vi "sim.vi"() -> ()   [LabVIEW 2011]
uses:
  <vilib>/robotics/Simulator/NI_Robotics_Simulator.lvlib
  <vilib>/robotics/Starter Kit/1.0/Sim Host Interface/NI_Robotics_Starter Kit Host_Sim_1.0.lvclass
  <vilib>/Analysis/NI_AALPro.lvlib
  <vilib>/Analysis/7linalg.llb/Real Transpose Matrix.vi
  <vilib>/Analysis/Matrix/NI_Matrix.lvlib
  <vilib>/robotics/Starter Kit/Host Interface/NI_Robotics_Starter Kit Host.lvclass
  <vilib>/Analysis/NI_AALBase.lvlib
  <vilib>/Platform/TimedLoop/XDataNode/XDataNode.xnode
  <vilib>/Platform/TimedLoop/XDataNode/timing_clust.ctl
  <vilib>/Platform/TimedLoop/XDataNode/XDNodeRunTimeDep.lvlib
  <vilib>/Platform/TimedLoop/XDataNode/wakeup.ctl
  <vilib>/Platform/TimedLoop/XDataNode/nitl_modes.ctl
  <vilib>/Analysis/baseanly.llb/Real A x B.vi
  <vilib>/Analysis/Matrix/Numeric/Conversions/Array To Matrix - RA.vi
panel:
  in  "q":dbl step=0.01
  in  "K_ W":dbl step=0.01
  in  "K_ VL":dbl step=0.01
  in  "Paso":dbl
  in  "Tiempo":dbl
  in  "stop":bool
  out "X-Y":cluster{ext[], ext[]}(graph)
  out "VL":cluster{i32[], dbl[]}(graph)
  out "W":cluster{i32[], dbl[]}(graph)
  out "theta":cluster{i32[], ext[]}(graph)
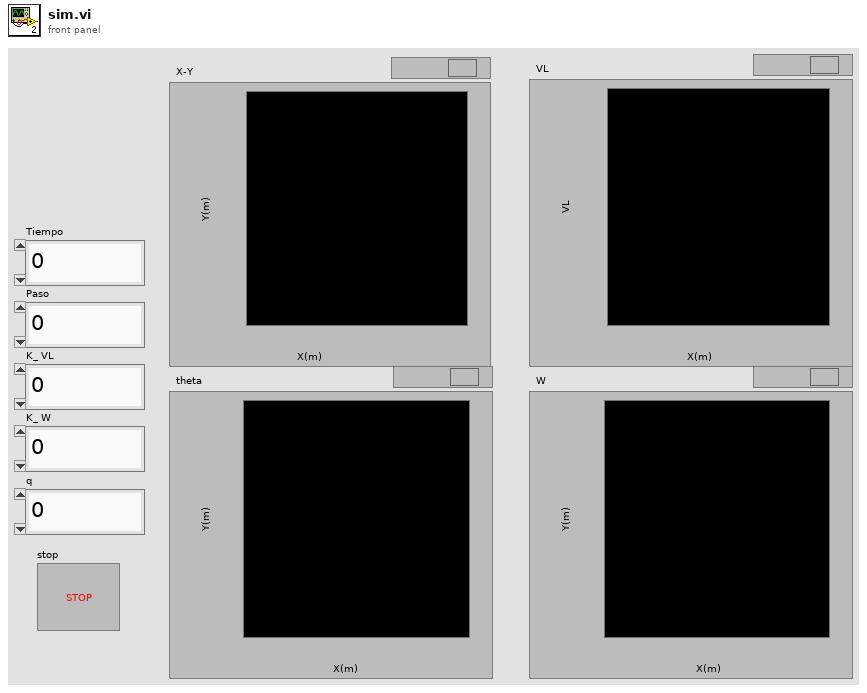
[diagram p1: front panel]
types:
  T1 = typedef "NI_Matrix.lvlib/RealMatrix.ctl" = dbl[][]
  T2 = typedef "XDNodeRunTimeDep.lvlib/timing_clust.ctl" = cluster{"Expected End [f-1]":u64, "Actual End [f-1]":u64, "Finished Late? [f-1]":bool, "Expected End [i-1]":u64, "Actual End [i-1]":u64, "Finished Late? [i-1]":bool, "Expected Start [i]":u64, "Actual Start [i]":u64, "Expected Start [f]":u64, "Actual Start [f]":u64, "Source Name":string, "Structure Name":string, "Period":i64, "Deadline":i64, "Offset":i64, "Start":i64, "Priority":i32, "Timeout":i32, "Mode":T3, "Wakeup Reason":T4, "Error":errorcluster, "Source Type":string, "Secondary Source Type":string, "Global End Time":u64, "Global Start Time":u64, "Frame Duration":u64, "Iteration Duration":u64, "Assigned CPU":i32, "I/O Scan Engine Mode":u32}
  T3 = typedef "XDNodeRunTimeDep.lvlib/nitl_modes.ctl" = enum32{"No Change", "Process missed periods, maintain original phase", "Discard missed periods, maintain original phase", "Process missed periods, ignore original phase", "Discard missed periods, ignore original phase"}
  T4 = typedef "XDNodeRunTimeDep.lvlib/wakeup.ctl" = enum32{"Normal", "Aborted", "Asynchronous wakeup", "Timing source error", "Timed loop error", "Timeout"}
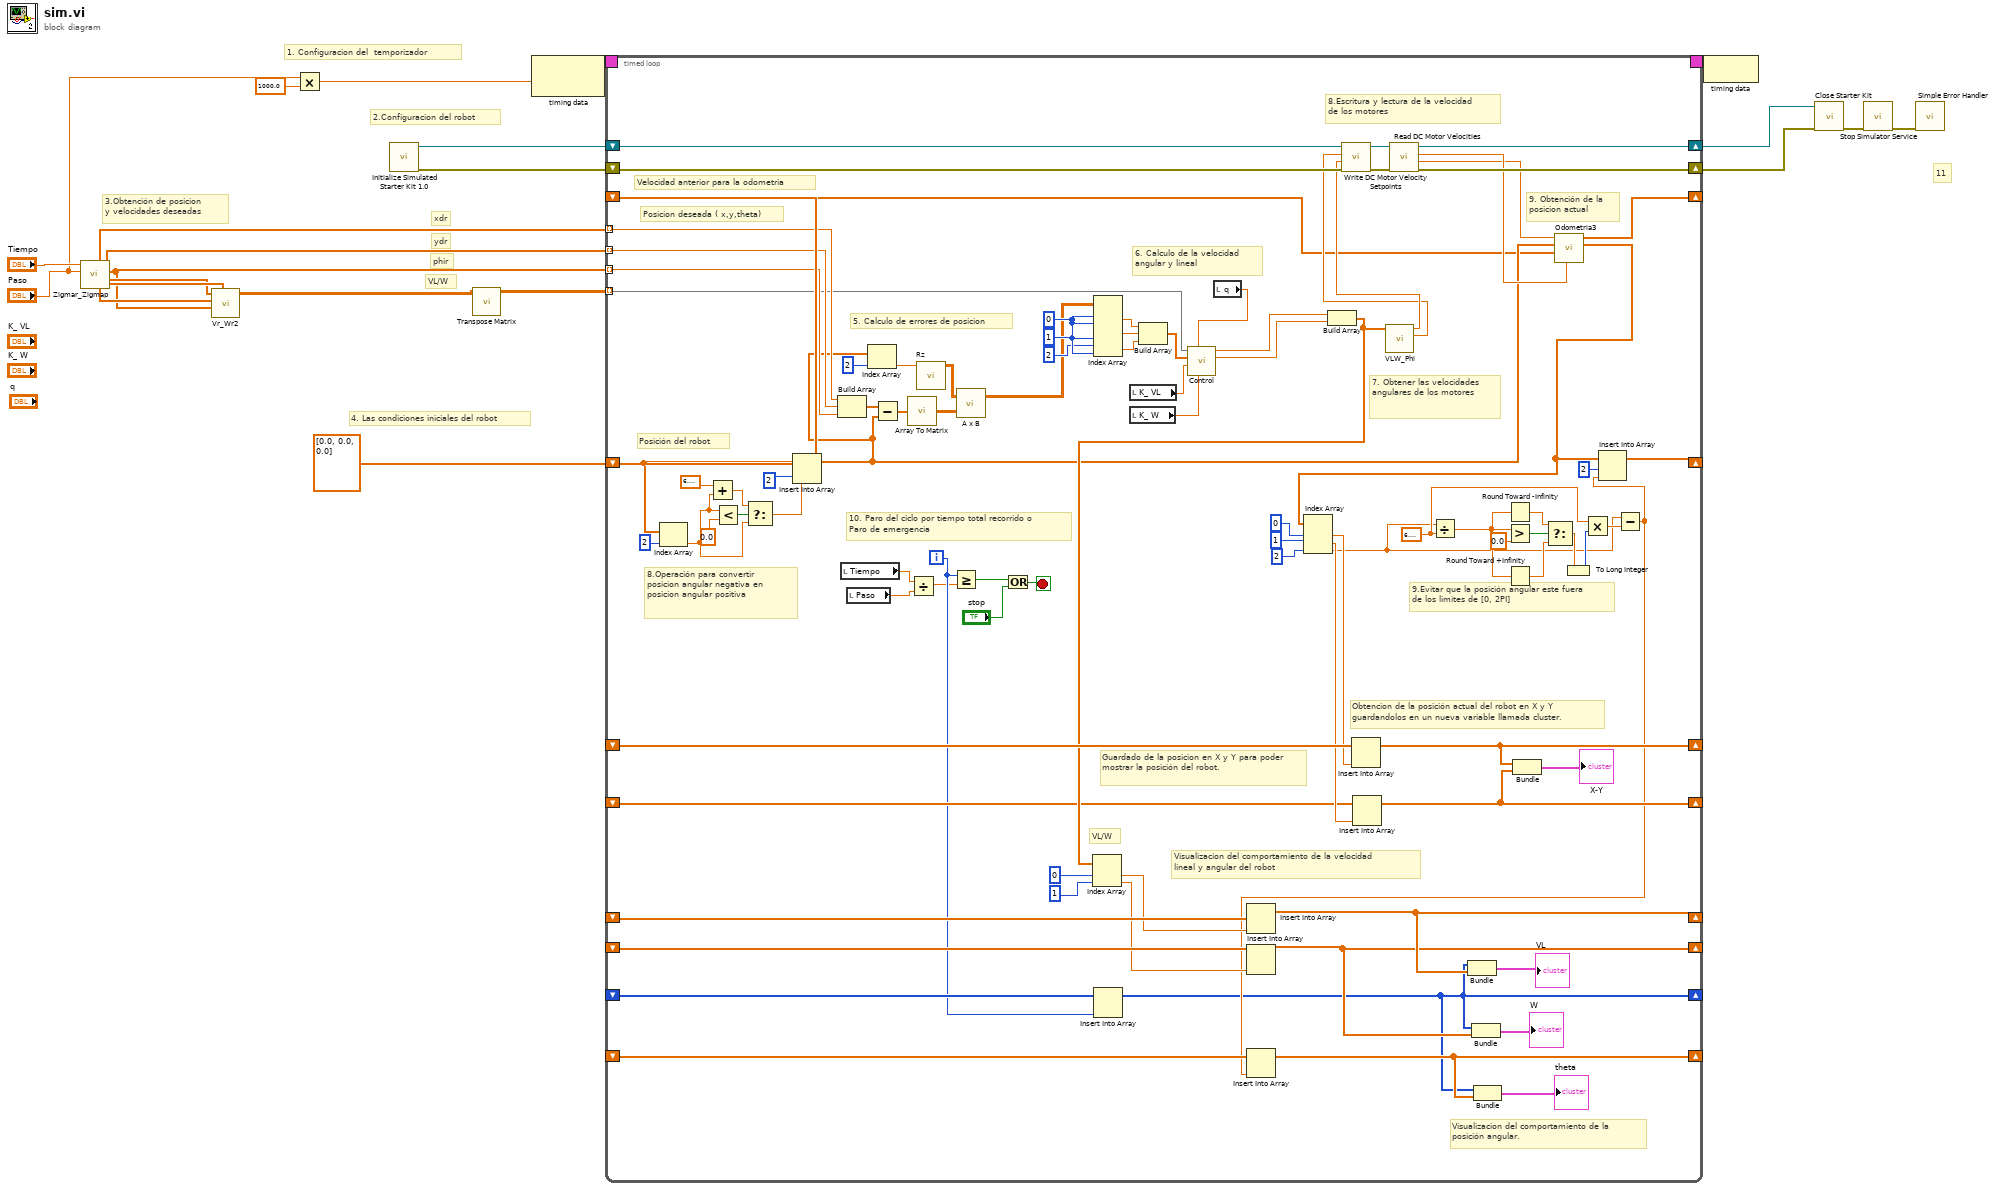
[diagram p0: block diagram]
diagram:
  w8 = dbl[] [0.0, 0.0, 0.0]
  # "4. Las condiciones iniciales del robot"
  # "VL/W"
  # "3.Obtención de posicion \ny velocidades deseadas"
  # "2.Configuracion del robot"
  # "1. Configuracion del  temporizador"
  # "phir"
  # "ydr"
  # "xdr"
  # "11"
  n1 = call "Zigmar_Zigmap.vi"("Paso"="Paso", "Tiempo"="Tiempo") -> ("Xdrp"=w16:dbl[], "Phir"=w14:dbl[], "Ydr"=w18:dbl[], "Ydrp"=w15:dbl[], "Xdr"=w13:dbl[], "Phirp"=w17:dbl[])  [unwired: 4 in]
  n2 = call "Vr_Wr2.vi"("Phirp"=w17, "Phir"=w14, "Ydrp"=w15, "Xdrp"=w16) -> ("VLW"=w2:T1)  [unwired: 7 in]
  n3 = Multiply(x="Paso", y=1000.0) -> (x*y=w5:dbl)
  n4 = call <vilib>:"Initialize Simulated Starter Kit 1.0.vi"() -> ("error out"=w4:errorcluster, "simulated starter kit host 1.0 out"=w3:refnum<class "NI_Robotics_Starter Kit Host_Sim_1.0.lvclass">)  [unwired: 10 in]
  n5 = call-poly <vilib>:"Transpose Matrix.vi"("Input Matrix"=w2) -> ("Matrix Transpose"=w1:T1)  [unwired: 9 in, 1 out]
  n6 = node-c288(w5) -> (w21:T2)
  n7 = timed-loop {
    shift-right: [w101] -> w9
    shift-left: w3 -> [w103]
    shift-right: [w100] -> w10
    shift-left: w4 -> [w102]
    timing: w21 -> [_]
    timing-out: [_] -> w20
    tunnel: w13 -> [w113] mode=indexing
    tunnel: w18 -> [w112] mode=indexing
    tunnel: w14 -> [w111] mode=indexing
    shift-right: [w89] -> _
    shift-left: w8 -> [w38]
    shift-right: [w37] -> _
    shift-left: w8 -> [w33]
    shift-right: [w93] -> _
    shift-left: _ -> [w98]
    shift-right: [w92] -> _
    shift-left: _ -> [w51]
    shift-right: [w68] -> _
    shift-left: _ -> [w77]
    shift-right: [w65] -> _
    shift-left: _ -> [w72]
    shift-right: [w62] -> _
    shift-left: _ -> [w67]
    shift-right: [w64] -> _
    shift-left: _ -> [w66]
    tunnel: w1 -> [w25] mode=indexing
    i -> [w50]
    stop <- w108 stop-if-true
    w60 = 0 ("index (col)")
    w88 = 6.283185307179586
    # "Visualizacion del comportamiento de la\nposición angular."
    # "Visualizacion del comportamiento de la velocidad \nlineal y angular del robot"
    # "VL/W"
    # "Obtencion de la posición actual del robot en X y Y\nguardandolos en un nueva variable llamada cluster."
    # "Guardado de la posicion en X y Y para poder mostrar la posición del robot."
    # "Posicion deseada ( x,y,theta)"
    # "10. Paro del ciclo por tiempo total recorrido o\nParo de emergencia"
    # "9.Evitar que la posición angular este fuera\nde los limites de [0, 2PI]"
    # "8.Operación para convertir posicion angular negativa en posicion angular positiva"
    # "Posición del robot"
    # "9. Obtención de la\nposicion actual"
    # "7. Obtener las velocidades\nangulares de los motores"
    # "6. Calculo de la velocidad \nangular y lineal"
    # "5. Calculo de errores de posicion"
    # "8.Escritura y lectura de la velocidad\nde los motores"
    # "Velocidad anterior para la odometria"
    n8 = Index Array(array=w38, index=2) -> (element=w41:ext)
    n9 = Add(x=6.283185307179586, y=w41) -> (x+y=w43:ext)
    n10 = Less?(x=w41, y=0.0) -> (x < y?=w46:bool)
    n11 = Select(t=w43, s=w46, f=w41) -> (s? t:f=w40:ext)
    n12 = Insert Into Array(array=w38, index=2, new element=w40) -> (w34:ext[])
    n13 = Build Array(w113, w112, w111) -> (w47:dbl[])
    n14 = local read "Tiempo"() -> (w27:dbl)
    n15 = local read "Paso"() -> (w28:dbl)
    n16 = Index Array(array=w34, index=2) -> (element=w110:ext)
    n17 = Subtract(x=w47, y=w34) -> (x-y=w106:ext[])
    n18 = call-poly <vilib>:"Array To Matrix.vi"("Real 1D Array"=w106) -> ("Real Matrix (Column Vector)"=w29:T1)
    n19 = Divide(x=w27, y=w28) -> (x/y=w26:dbl)
    n20 = call "Rz.vi"("theta"=w110) -> ("RotacionalZ"=w30:T1)  [unwired: 10 in]
    n21 = Greater Or Equal?(x=w50, y=w26) -> (x >= y?=w99:bool)
    n22 = call-poly <vilib>:"A x B.vi"("B"=w29, "A"=w30) -> ("A x B"=w31:T1)  [unwired: 1 out]
    n23 = Or(x=w99, y="stop") -> (x .or. y?=w108:bool)
    n24 = Index Array(array=w31, index (row) #1=w60, index (col) #1=w60, index (row) #2=1 ("index (row)"), index (col) #2=w60, index (row) #3=2 ("index (row)"), index (col) #3=w60) -> (element #1=w57:dbl, element #2=w56:dbl, element #3=w55:dbl)
    n25 = Insert Into Array(array=w67, new element=w50) -> (w62:i32[])  [unwired: 1 in]
    n26 = local read "K_ VL"() -> (w24:dbl)
    n27 = local read "K_ W"() -> (w23:dbl)
    n28 = Build Array(w57, w56, w55) -> (w54:dbl[])
    n29 = local read "q"() -> (w22:dbl)
    n30 = call "Control.vi"("Kp2"=w23, "Q"=w22, "KV"=w24, "Zigmae"=w54, "Vr/Wr"=w25) -> ("W"=w52:dbl, "V"=w53:dbl)  [unwired: 5 in]
    n31 = Build Array(w53, w52) -> (w76:dbl[])
    n32 = Index Array(array=w76, index #1=0 ("index"), index #2=1 ("index")) -> (element #1=w73:dbl, element #2=w71:dbl)
    n33 = Insert Into Array(array=w77, new element=w73) -> (w68:dbl[])  [unwired: 1 in]
    n34 = Insert Into Array(array=w72, new element=w71) -> (w65:dbl[])  [unwired: 1 in]
    n35 = call "VLW_Phi.vi"("VL/W"=w76) -> ("PhiL"=w48:dbl, "PhiR"=w49:dbl)  [unwired: 9 in]
    n36 = call <vilib>:"Write DC Motor Velocity Setpoints.vi"("error in (no error)"=w102, "right motor ccw velocity (rad/s)"=w49, "left motor ccw velocity (rad/s)"=w48, "starter kit host in"=w103) -> ("error out"=w105:errorcluster, "starter kit host out"=w104:refnum<class "NI_Robotics_Starter Kit Host_Sim_1.0.lvclass">)  [unwired: 6 in]
    n37 = call <vilib>:"Read DC Motor Velocities.vi"("error in (no error)"=w105, "starter kit host in"=w104) -> ("error out"=w100:errorcluster, "right motor ccw velocity (rad/s)"=w32:dbl, "left motor ccw velocity (rad/s)"=w35:dbl, "starter kit host out"=w101:refnum<class "NI_Robotics_Starter Kit Host_Sim_1.0.lvclass">)  [unwired: 6 in]
    n38 = Bundle(w62, w68) -> (→"VL":cluster{i32[], dbl[]})  [unwired: 1 in]
    n39 = Bundle(w62, w65) -> (→"W":cluster{i32[], dbl[]})  [unwired: 1 in]
    n40 = call "Odometria3.vi"("left motor ccw velocity (rad/s)"=w35, "Arrastrado"=w33, "Zigma"=w34, "right motor ccw velocity (rad/s)"=w32) -> ("Posicion estimada"=w36:ext[], "Velocidad actual"=w37:dbl[])  [unwired: 6 in]
    n41 = Index Array(array=w36, index #1=0 ("index"), index #2=1 ("index"), index #3=2 ("index")) -> (element #1=w95:ext, element #2=w94:ext, element #3=w79:ext)
    n42 = Insert Into Array(array=w98, new element=w95) -> (w93:ext[])  [unwired: 1 in]
    n43 = Insert Into Array(array=w51, new element=w94) -> (w92:ext[])  [unwired: 1 in]
    n44 = Divide(x=w79, y=w88) -> (x/y=w83:ext)
    n45 = Round Toward -Infinity(1:w83) -> (0:w85:ext)
    n46 = Greater?(x=w83, y=0.0) -> (0:w87:bool)
    n47 = Round Toward +Infinity(x=w83) -> (ceil(x): smallest int >= x=w82:ext)
    n48 = Bundle(w93, w92) -> (→"X-Y":cluster{ext[], ext[]})  [unwired: 1 in]
    n49 = Select(t=w85, s=w87, f=w82) -> (s? t:f=w80:ext)
    n50 = To Long Integer(number=w80) -> (32bit integer=w81:i32)
    n51 = Multiply(x=w88, y=w81) -> (x*y=w86:dbl)
    n52 = Subtract(x=w79, y=w86) -> (x-y=w63:ext)
    n53 = Insert Into Array(array=w66, new element=w63) -> (w64:ext[])  [unwired: 1 in]
    n54 = Bundle(w62, w64) -> (→"theta":cluster{i32[], ext[]})  [unwired: 1 in]
    n55 = Insert Into Array(array=w36, index=2, new element=w63) -> (w89:ext[])
  }
  n56 = node-c288(w20) -> ()
  n57 = call-dynamic "Close Starter Kit.vi"("error in (no error)"=w10, "starter kit host in"=w9) -> ("error out"=w12:errorcluster)  [unwired: 9 in]
  n58 = call <vilib>:"Stop Simulator Service.vi"("error in (no error)"=w12) -> ("error out"=w11:errorcluster)  [unwired: 10 in]
  n59 = call <vilib>:"Simple Error Handler.vi"("error in (no error)"=w11) -> ()  [unwired: 4 in, 5 out]
